vi "Get Image Data All Channels.vi"(6 "serial channels":string[](array[string]), 8 "error in (no error)":errorcluster, 9 "raw display notifier":refnum<notifier>, 10 "'stop' notifier":refnum<notifier>, 11 "fpga interface in":refnum<k20>) -> (0 "error out":errorcluster)   [LabVIEW 2026]
uses:
  Types/Serial Channel Display Parameters.ctl
  <vilib>/vision/Image Controls.llb/IMAQ Image.ctl
  Types/RAW Interpretation for Display.ctl
  GettingStarted_Common_148X_Host.lvlib
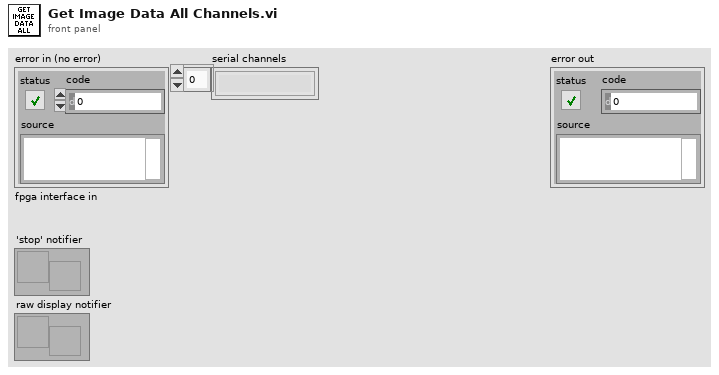
[diagram p1: front panel]
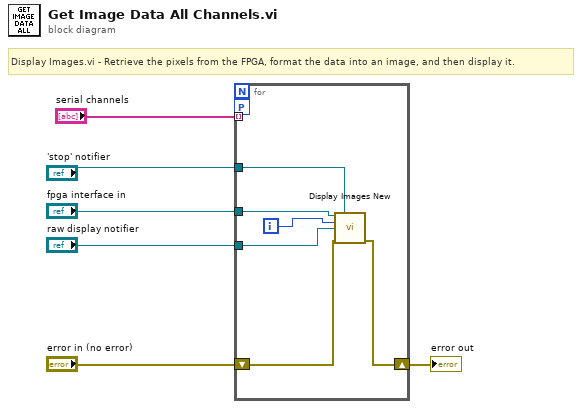
[diagram p0: block diagram]
diagram:
  # "Display Images.vi - Retrieve the pixels from the FPGA, format the data into an image, and then display it."
  n1 = for {
    tunnel: "fpga interface in" -> [w8]
    shift-right: [w12] -> w5
    shift-left: "error in (no error)" -> [w11]
    tunnel: "'stop' notifier" -> [w7]
    tunnel: "raw display notifier" -> [w10]
    tunnel: "serial channels" -> [_] mode=indexing
    workers-P: _ -> [_]
    i -> [w9]
    n2 = call "Display Images New.vi"("fpga interface in"=w8, "'stop' notifier"=w7, "display channel number"=w9, "raw display notifier"=w10, "error in (no error)"=w11) -> ("error out"=w12:errorcluster)  [unwired: 9 in, 1 out]
  }
  "error out" <- w5
